vi "DSF.Engine.Debug Flags.Set FIFO Flags.vi"(10 "FIFO":refnum<class "DSF.Engine.Debug Flags.FIFO.lvclass">, 11 "Debug Flags in":refnum<class "DSF.Engine.Debug Flags.lvclass">) -> (3 "Debug Flags out":refnum<class "DSF.Engine.Debug Flags.lvclass">)   [LabVIEW 2017, in "Data Sharing Framework Engine.lvlib" / "DSF.Engine.Debug Flags.lvclass"]
uses:
  DSF.Engine.Debug Flags.lvclass
  DSF.Engine.Debug Flags.FIFO.lvclass
  DSF.Engine.Debug Flags.lvclass/DSF.Engine.Debug Flags.ctl
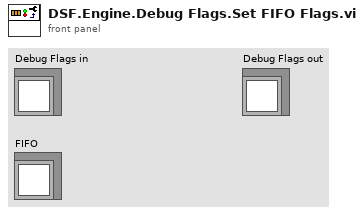
[diagram p1: front panel]
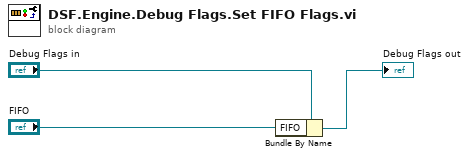
[diagram p0: block diagram]
diagram:
  n1 = Bundle By Name(cluster="Debug Flags in", "FIFO"="FIFO") -> (→"Debug Flags out":refnum<class "DSF.Engine.Debug Flags.lvclass">)
